vi "Stop.vi"(8 "error in (no error)":errorcluster caption="错误输入（无错误）", 11 "Execute 输入":refnum<class "Execute.lvclass">) -> (0 "error out":errorcluster caption="错误输出", 3 "Execute 输出":refnum<class "Execute.lvclass">)   [LabVIEW 2018, in "QMH_Class.lvlib" / "TestManager.lvlib" / "Execute.lvclass"]
uses:
  Execute.lvclass
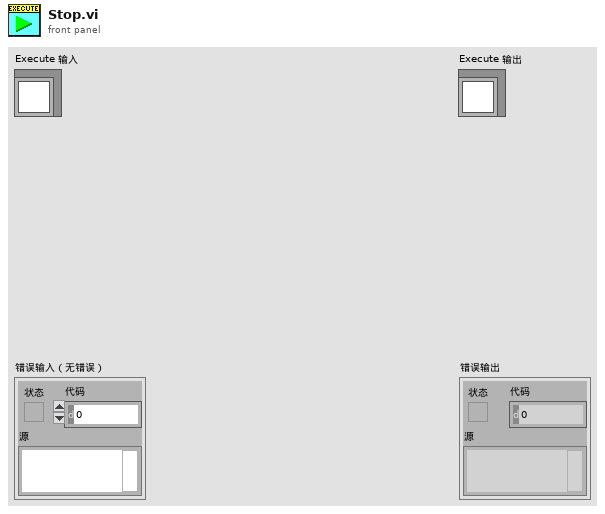
[diagram p1: front panel]
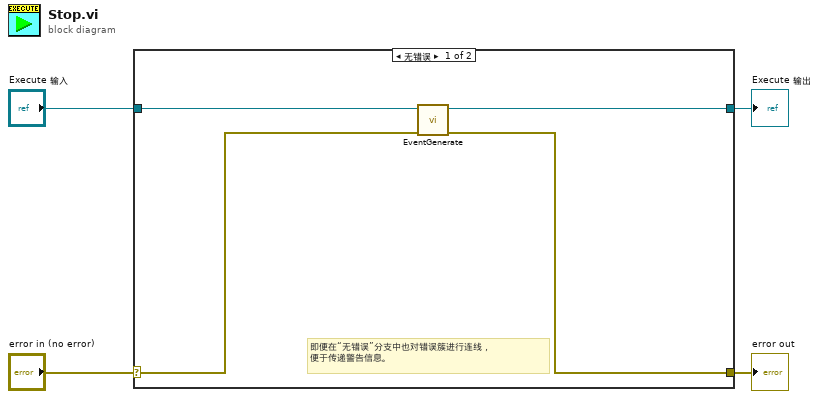
[diagram p0: block diagram]
diagram:
  n1 = case shown="无错误" "error in (no error)" {
    selector: "error in (no error)" -> [w6 w10]
    tunnel: [w5 w10] -> w3
    tunnel: [w7 w9] -> w1
    tunnel: "Execute 输入" -> [w8 w9]
    frame No Error {
      # "即便在“无错误”分支中也对错误簇进行连线，\n便于传递警告信息。"
      n2 = call "EventGenerate.vi"("error in (no error)"=w6, "Execute"=w8) -> ("error out"=w5:errorcluster, "Execute"=w7:refnum<class "Execute.lvclass">)  [unwired: 8 in]
    }
    frame Error {
    }
  }
  "error out" <- w3
  "Execute 输出" <- w1
